vi "GetTag.vi"(8 "default":string, 10 "tag":string, 11 "String in":string) -> (0 "Exists?":bool, 1 "after tag":string, 2 "body":string, 3 "before tag":string)   [LabVIEW 2020]
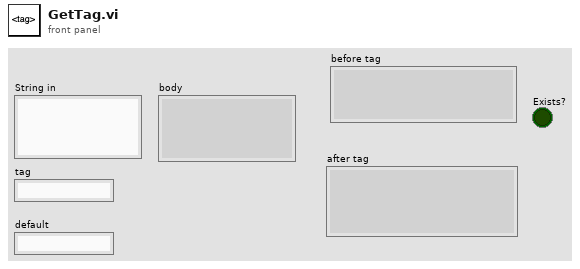
[diagram p1: front panel]
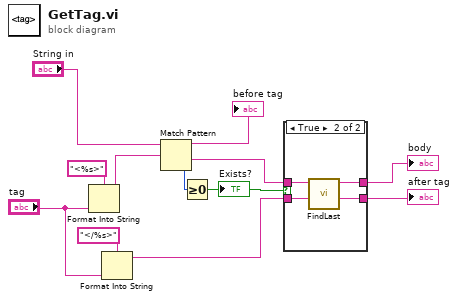
[diagram p0: block diagram]
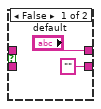
[diagram p2: hidden frame]
diagram:
  n1 = Format Into String(format string="<%s>", "tag") -> (resulting string=w8:string)  [unwired: 2 in, 1 out]
  n2 = Format Into String(format string="</%s>", "tag") -> (resulting string=w4:string)  [unwired: 2 in, 1 out]
  n3 = Match Pattern(string="String in", regular expression=w8) -> (before substring=→"before tag":string, after substring=w11:string, offset past match=w2:i32)  [unwired: 1 in, 1 out]
  n4 = Greater Or Equal To 0?(x=w2) -> (x >= 0?=w1:bool)
  "Exists?" <- w1
  n5 = case shown="True" w1 {
    tunnel: ["default" w18] -> w12
    tunnel: w11 -> [_ w17]
    tunnel: w4 -> [_ w16]
    tunnel: ["" ("after") w15] -> w3
    frame False {
    }
    frame True {
      n6 = call "FindLast.vi"("pattern"=w16, "String"=w17) -> ("after"=w15:string, "before"=w18:string)  [unwired: 8 in]
    }
  }
  "body" <- w12
  "after tag" <- w3
